vi "Generate Sine.vi"(4 "Error In":errorcluster, 5 "Numeric":i32) -> (0 "Error Out":errorcluster, 2 "Sine":dbl)   [LabVIEW 2012]
doc: "This VI generates a Sine Wave one point at a time."
uses:
  <vilib>/ptbypt/NI_PtbyPt.lvlib
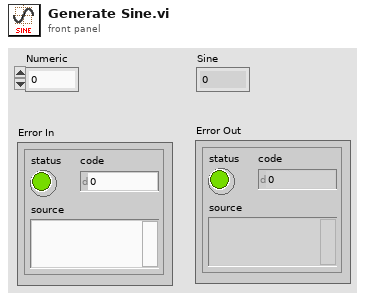
[diagram p1: front panel]
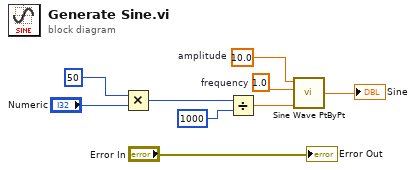
[diagram p0: block diagram]
diagram:
  w4 = 1.0  # frequency
  w3 = 10.0  # amplitude
  n1 = Multiply(x=u32 50 ("milliseconds to wait"), y="Numeric") -> (x*y=w8:u32)
  n2 = Divide(x=w8, y=u32 1000) -> (x/y=w9:dbl)
  n3 = call <vilib>:"Sine Wave PtByPt.vi"("time"=w9, "frequency"=w4, "amplitude"=w3) -> ("sine wave"=→"Sine":dbl)  [unwired: 1 in]
  "Error Out" <- "Error In"
